vi "show_hypertables.vi"(7 "connection_reference":T1, 8 "error in (no error)":errorcluster) -> (0 "error out":errorcluster, 3 "hyper_table_names []":string[](array[string]))   [LabVIEW 2015, in "lv-timescaledb.lvlib"]
uses:
  lv-timescaledb.lvlib
  <vilib>/addons/database/Connection.llb/Conn ObjectReference.ctl
  <vilib>/addons/database/Command.llb/Cmd Execute.vi
  <vilib>/addons/database/Recordset.llb/Rec Fetch Recordset Data (CR).vi
  <vilib>/addons/database/Recordset.llb/Rec Destroy - Command.vi
  <vilib>/addons/database/Command.llb/Cmd Delete.vi
  <vilib>/addons/database/NI_Database_API.lvlib
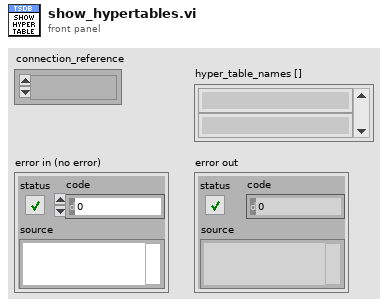
[diagram p1: front panel]
types:
  T1 = typedef "NI_Database_API.lvlib/Conn ObjectReference.ctl" = refnum<k1>
  T2 = typedef "NI_Database_API.lvlib/Cmd ObjectReference.ctl" = refnum<k1>
  T3 = typedef "NI_Database_API.lvlib/Cmd-Rec Object Reference.ctl" = refnum<k1>
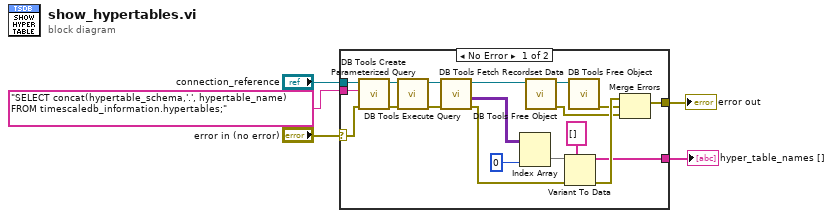
[diagram p0: block diagram]
diagram:
  n1 = case shown="No Error" "error in (no error)" {
    selector: "error in (no error)" -> [w6 w25]
    tunnel: "connection_reference" -> [w15 _]
    tunnel: [w24 w25] -> w3
    tunnel: [w9 _] -> w1
    tunnel: "SELECT concat(hypertable_schema,'.', hypertable_name) FROM timescaledb_information.hypertables;" -> [w14 _]
    frame No Error {
      n2 = call <vilib>:"DB Tools Create Parameterized Query.vi"("error in (no error)"=w6, "SQL query"=w14, "connection reference"=w15) -> ("error out"=w18:errorcluster, "command reference"=w19:T2)  [unwired: 4 in, 1 out]
      n3 = call-poly <vilib>:"DB Tools Execute Query.vi"("error in (no error)"=w18, "command reference"=w19) -> ("error out"=w13:errorcluster, "command-recordset reference"=w16:T3)  [unwired: 6 in]
      n4 = call-poly <vilib>:"DB Tools Fetch Recordset Data.vi"("error in (no error)"=w13, "command-recordset reference"=w16) -> ("error out"=w23:errorcluster, "recordset data"=w21:variant[][], "command-recordset reference out"=w17:T3)  [unwired: 3 in]
      n5 = Index Array(array=w21, index (col)=0 ("disabled index (col)")) -> (element=w10:variant[])  [unwired: 1 in]
      n6 = call-poly <vilib>:"DB Tools Free Object.vi"("command-recordset reference"=w17) -> ("error out"=w11:errorcluster, "command reference"=w20:T2)  [unwired: 9 in]
      n7 = Variant To Data(error in=w23, type=string[] [], Variant=w10) -> (data=w9:string[], error out=w22:errorcluster)
      n8 = call-poly <vilib>:"DB Tools Free Object.vi"("command reference"=w20) -> ("error out"=w12:errorcluster)  [unwired: 9 in, 1 out]
      n9 = Merge Errors(w22, w12, w11) -> (w24:errorcluster)
    }
    frame Error {
    }
  }
  "error out" <- w3
  "hyper_table_names []" <- w1
